vi "BuildCall.vi"(7 "PythonConverter_BD in":refnum<class "PyConvBD.lvclass">, 8 "error in":errorcluster, 11 "DiagramDisable in":refnum<class "DiagramDisable.lvclass">) -> (0 "error out":errorcluster, 3 "DiagramDisable out":refnum<class "DiagramDisable.lvclass">, 5 "PythonConverter_BD out":refnum<class "PyConvBD.lvclass">)   [LabVIEW 2014, in "Raspberry Pi Compatible Compiler for LabVIEW.lvlib" / "DiagramDisable.lvclass"]
uses:
  DiagramDisable.lvclass
  Python/PythonConverter_BD/PyConvBD.lvclass
  Python/Parsing/ListTypesTD.ctl
  Python/PythonConverter_BD/TypeDefs/NodeCall_TD.ctl
  Tunnel/Tunnel.lvclass
  Python/Parsing/Python Functions.lvlib
  Raspberry Pi Compatible Compiler for LabVIEW.lvlib
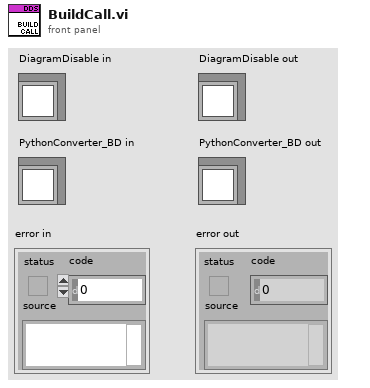
[diagram p1: front panel]
types:
  T1 = typedef "Raspberry Pi Compatible Compiler for LabVIEW.lvlib/NodeCall_TD.ctl" = cluster{"call":string, "collect":string, "Threaded":bool, "branches":string[]}
  T2 = typedef "Raspberry Pi Compatible Compiler for LabVIEW.lvlib/Python Functions.lvlib/ListTypesTD.ctl" = enum16{"list", "tuple", "parameter list", "output list", "return values"}
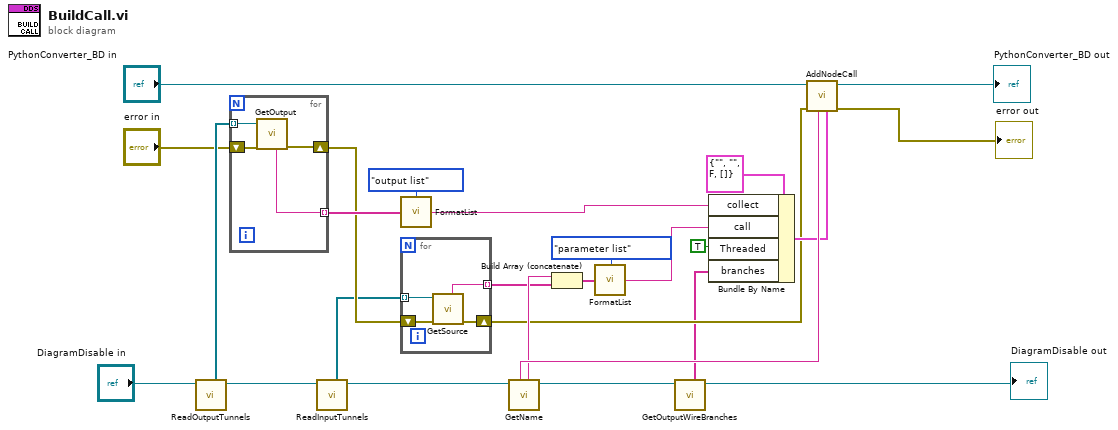
[diagram p0: block diagram]
diagram:
  n1 = call-dynamic "ReadOutputTunnels.vi"("Structure in"="DiagramDisable in") -> ("Structure out"=w21:refnum<class "DiagramDisable.lvclass">, "outputs"=w22:refnum<class "Tunnel.lvclass">[])  [unwired: 7 in]
  n2 = for {
    tunnel: w22 -> [w30] mode=indexing
    shift-right: [w27] -> w20
    shift-left: "error in" -> [w29]
    tunnel: [w28] -> w26 mode=indexing
    n3 = call-dynamic "GetOutput.vi"("error in"=w29, "Tunnel in"=w30) -> ("error out"=w27:errorcluster, "name"=w28:string)  [unwired: 5 in, 1 out]
  }
  n4 = call-dynamic "ReadInputTunnels.vi"("Structure in"=w21) -> ("Structure out"=w18:refnum<class "DiagramDisable.lvclass">, "tunnels"=w19:refnum<class "Tunnel.lvclass">[])  [unwired: 7 in]
  n5 = call "FormatList.vi"("values"=w26, "type"=ListTypesTD."output list") -> ("python object"=w16:string)
  n6 = for {
    tunnel: w19 -> [w34] mode=indexing
    shift-right: [w32] -> w11
    shift-left: w20 -> [w33]
    tunnel: [w31] -> w13 mode=indexing
    n7 = call-dynamic "GetSource.vi"("error in"=w33, "Tunnel in"=w34) -> ("error out"=w32:errorcluster, "name"=w31:string)  [unwired: 5 in, 1 out]
  }
  n8 = call-dynamic "GetName.vi"("Structure in"=w18) -> ("Structure out"=w8:refnum<class "DiagramDisable.lvclass">, "name"=w14:string, "UID"=w23:string)  [unwired: 5 in, 1 out]
  n9 = Build Array (concatenate)(w14, w13) -> (w12:string[])
  n10 = call "FormatList.vi"("values"=w12, "type"=ListTypesTD."parameter list") -> ("python object"=w10:string)
  n11 = call-dynamic "GetOutputWireBranches.vi"("Structure in"=w8) -> ("Structure out"=→"DiagramDisable out":refnum<class "DiagramDisable.lvclass">, "branches"=w7:string[])  [unwired: 6 in, 1 out]
  n12 = Bundle By Name(cluster=T1 {"call"="", "collect"="", "Threaded"=FALSE, "branches"=[]} ("call"), "collect"=w16, "call"=w10, "Threaded"=TRUE, "branches"=w7) -> (w15:T1)
  n13 = call "AddNodeCall.vi"("call"=w15, "name"=w23, "error in"=w11, "PythonConverter_BD in"="PythonConverter_BD in") -> ("error out"=→"error out":errorcluster, "PythonConverter_BD out"=→"PythonConverter_BD out":refnum<class "PyConvBD.lvclass">)  [unwired: 4 in]
